vi "脉冲测量_基于频率_有限.vi"() -> ()   [LabVIEW 2013]
uses:
  <userlib>/ArtDAQ/_SubVI/ArtDAQ_CreateCIPulseChanFreq.vi
  <userlib>/ArtDAQ/_SubVI/ArtDAQ_CfgImplicitTiming.vi
  <userlib>/ArtDAQ/_SubVI/ArtDAQ_Read Counter Freq NSamp.vi
panel:
  out "占空比":dbl[](array[numeric])
  in  "每通道点数":i32=1000
  in  "Stop":bool
  out "频率":dbl[](array[numeric])
  in  "计数器":string="Dev1/ctr0"
  in  "最小值":dbl=0.1 format="%0.6f"
  in  "MaxValue":dbl=2000000.0 caption="最大值" format="%0.6f"
  out "错误输出":errorcluster
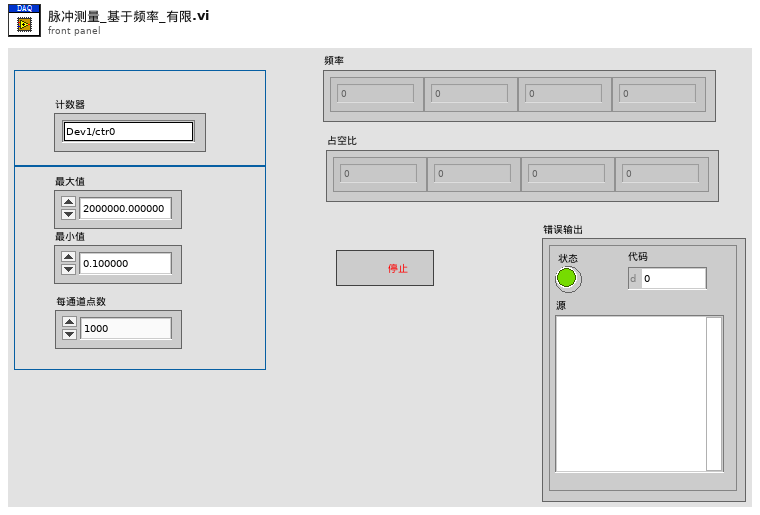
[diagram p1: front panel]
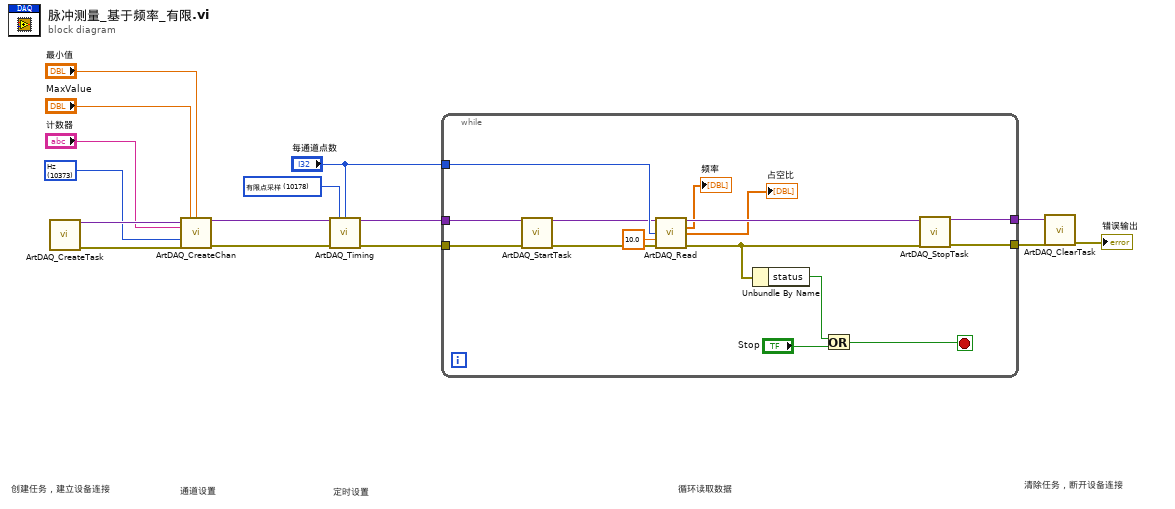
[diagram p0: block diagram]
diagram:
  w1 = 10373 items=["Hz"=10373] ("Units")
  w5 = 10178 items=["有限点采样"=10178, "连续采样"=10123] ("SampleMode")
  # "清除任务，断开设备连接"
  # "循环读取数据"
  # "定时设置"
  # "通道设置"
  # "创建任务，建立设备连接"
  n1 = call <userlib>:"ArtDAQ_CreateTask.vi"() -> ("任务句柄"=w15:variant, "错误输出"=w14:errorcluster)  [unwired: 14 in]
  n2 = call-poly <userlib>:"ArtDAQ_CreateChan.vi"("任务句柄"=w15, "最大值"="MaxValue", "最小值"="最小值", "计数器"="计数器", "单位"=w1, "错误输入"=w14) -> ("任务句柄"=w7:variant, "错误输出"=w6:errorcluster)  [unwired: 8 in]
  n3 = call-poly <userlib>:"ArtDAQ_Timing.vi"("任务句柄"=w7, "采样模式"=w5, "每通道采样数"="每通道点数", "错误输入"=w6) -> ("任务句柄"=w3:variant, "错误输出"=w2:errorcluster)  [unwired: 10 in]
  n4 = while {
    tunnel: [w29] -> w12
    tunnel: [w27] -> w11
    tunnel: "每通道点数" -> [w26]
    tunnel: w3 -> [w25]
    tunnel: w2 -> [w24]
    stop <- w16 stop-if-true
    n5 = call <userlib>:"ArtDAQ_StartTask.vi"("任务句柄"=w25, "错误输入"=w24) -> ("任务句柄"=w23:variant, "错误输出"=w22:errorcluster)  [unwired: 12 in]
    n6 = call-poly <userlib>:"ArtDAQ_Read.vi"("任务句柄"=w23, "每通道采样数"=w26, "超时s"=10.0 ("Timeout"), "错误输入"=w22) -> ("任务句柄"=w30:variant, "频率"=→"频率":dbl[], "占空比"=→"占空比":dbl[], "错误输出"=w28:errorcluster)  [unwired: 8 in]
    n7 = Unbundle By Name(w28) -> ("status"=w19:bool)
    n8 = Or(x=w19, y="Stop") -> (x .or. y?=w16:bool)
    n9 = call <userlib>:"ArtDAQ_StopTask.vi"("任务句柄"=w30, "错误输入"=w28) -> ("任务句柄"=w29:variant, "错误输出"=w27:errorcluster)  [unwired: 12 in]
  }
  n10 = call <userlib>:"ArtDAQ_ClearTask.vi"("任务句柄"=w12, "错误输入"=w11) -> ("错误输出"=→"错误输出":errorcluster)  [unwired: 13 in]
